vi "DisplayJson.vi"(11 "JSON String In":string="[{\"version\":\"1.0.0\",\"header\":{\"creationDate\":\"2022-06-03T00:00:00\",\"remarks\":\"\",\"serialNumber\":\"98172\",\"productNumber\":\"123021.1804\",\"productType\":\"PAA-9L\",\"pressureType\":2,\"productSeries\":\"9L\",\"compensatedTemperatureRange\":{\"min\":-10.0,\"max\":80.0,\"unit\":4},\"compensatedPressureRange\":{\"min\":0.0,\"max\":0.35,\"unit\":3},\"electricSupply\":{\"magnitude\":1.0,\"unit\":18},\"orderNumber\":9990266,\"orderPosition\":3,\"orderTargetDispatchDate\":\"2022-06-02T00:00:00+00:00\",\"customerName\":\"DemoData Inc.\",\"customerNumber\":12345678,\"customerOrderNumber\":\"Cust-9990266-123\",\"customerReferenceNumber\":\"\",\"customerProductT...") -> ()   [LabVIEW 2017] (continued)
output\":{\"magnitude\":0.109965,\"unit\":3},\"error\":{\"magnitude\":-0.0092906517,\"unit\":7}},\"temperature\":{\"output\":{\"magnitude\":19.5444,\"unit\":4},\"error\":{\"magnitude\":-0.0064905507,\"unit\":4}}}}}},{\"reference\":\"F_12300_XX_0000098765\",\"environmentTarget\":{\"pressure\":{\"magnitude\":0.19,\"unit\":3},\"temperature\":{\"magnitude\":20.0,\"unit\":4}},\"environment\":{\"pressure\":{\"magnitude\":0.190006,\"unit\":3},\"temperature\":{\"magnitude\":19.5509,\"unit\":4},\"supply\":{\"magnitude\":1.0,\"unit\":18}},\"raw\":{\"signal\":{\"magnitude\":42.078711244,\"unit\":22},\"bridgeResistance\":{\"magnitude\":3496.1789897,\"unit\":28}},\"compensated\":{\"mathematicalModels\":{\"MM0123\":{\"pressure\":{\"output\":{\"magnitude\":0.190012,\"unit\":3},\"error\":{\"magnitude\":0.0015735789,\"unit\":7}},\"temperature\":{\"output\":{\"magnitude\":19.544,\"unit\":4},\"error\":{\"magnitude\":-0.0068909382,\"unit\":4}}}}}},{\"reference\":\"F_12300_XX_0000098765\",\"environmentTarget\":{\"pressure\":{\"magnitude\":0.27,\"unit\":3},\"temperature\":{\"magnitude\":20.0,\"unit\":4}},\"environment\":{\"pressure\":{\"magnitude\":0.269992,\"unit\":3},\"temperature\":{\"magnitude\":19.5509,\"unit\":4},\"supply\":{\"magnitude\":1.0,\"unit\":18}},\"raw\":{\"signal\":{\"magnitude\":54.069872892,\"unit\":22},\"bridgeResistance\":{\"magnitude\":3491.6914255,\"unit\":28}},\"compensated\":{\"mathematicalModels\":{\"MM0123\":{\"pressure\":{\"output\":{\"magnitude\":0.27003,\"unit\":3},\"error\":{\"magnitude\":0.010759802,\"unit\":7}},\"temperature\":{\"output\":{\"magnitude\":19.5372,\"unit\":4},\"error\":{\"magnitude\":-0.013679718,\"unit\":4}}}}}},{\"reference\":\"F_12300_XX_0000098765\",\"environmentTarget\":{\"pressure\":{\"magnitude\":0.35,\"unit\":3},\"temperature\":{\"magnitude\":20.0,\"unit\":4}},\"environment\":{\"pressure\":{\"magnitude\":0.350007,\"unit\":3},\"temperature\":{\"magnitude\":19.5509,\"unit\":4},\"supply\":{\"magnitude\":1.0,\"unit\":18}},\"raw\":{\"signal\":{\"magnitude\":66.008929835,\"unit\":22},\"bridgeResistance\":{\"magnitude\":3487.3457136,\"unit\":28}},\"compensated\":{\"mathematicalModels\":{\"MM0123\":{\"pressure\":{\"output\":{\"magnitude\":0.350006,\"unit\":3},\"error\":{\"magnitude\":-0.00038101157,\"unit\":7}},\"temperature\":{\"output\":{\"magnitude\":19.5357,\"unit\":4},\"error\":{\"magnitude\":-0.015189517,\"unit\":4}}}}}},{\"reference\":\"F_12300_XX_0000098765\",\"environmentTarget\":{\"pressure\":{\"magnitude\":0.03,\"unit\":3},\"temperature\":{\"magnitude\":40.0,\"unit\":4}},\"environment\":{\"pressure\":{\"magnitude\":0.0299915,\"unit\":3},\"temperature\":{\"magnitude\":39.7284,\"unit\":4},\"supply\":{\"magnitude\":1.0,\"unit\":18}},\"raw\":{\"signal\":{\"magnitude\":19.022094163,\"unit\":22},\"bridgeResistance\":{\"magnitude\":3681.6183819,\"unit\":28}},\"compensated\":{\"mathematicalModels\":{\"MM0123\":{\"pressure\":{\"output\":{\"magnitude\":0.0300123,\"unit\":3},\"error\":{\"magnitude\":0.0059539043,\"unit\":7}},\"temperature\":{\"output\":{\"magnitude\":39.719,\"unit\":4},\"error\":{\"magnitude\":-0.0093796899,\"unit\":4}}}}}},{\"reference\":\"F_12300_XX_0000098765\",\"environmentTarget\":{\"pressure\":{\"magnitude\":0.11,\"unit\":3},\"temperature\":{\"magnitude\":40.0,\"unit\":4}},\"environment\":{\"pressure\":{\"magnitude\":0.110003,\"unit\":3},\"temperature\":{\"magnitude\":39.7284,\"unit\":4},\"supply\":{\"magnitude\":1.0,\"unit\":18}},\"raw\":{\"signal\":{\"magnitude\":31.15514702,\"unit\":22},\"bridgeResistance\":{\"magnitude\":3676.9975385,\"unit\":28}},\"compensated\":{\"mathematicalModels\":{\"MM0123\":{\"pressure\":{\"output\":{\"magnitude\":0.109971,\"unit\":3},\"error\":{\"magnitude\":-0.0090594959,\"unit\":7}},\"temperature\":{\"output\":{\"magnitude\":39.7198,\"unit\":4},\"error\":{\"magnitude\":-0.0086481985,\"unit\":4}}}}}},{\"reference\":\"F_12300_XX_0000098765\",\"environmentTarget\":{\"pressure\":{\"magnitude\":0.19,\"unit\":3},\"temperature\":{\"magnitude\":40.0,\"unit\":4}},\"environment\":{\"pressure\":{\"magnitude\":0.190008,\"unit\":3},\"temperature\":{\"magnitude\":39.7284,\"unit\":4},\"supply\":{\"magnitude\":1.0,\"unit\":18}},\"raw\":{\"signal\":{\"magnitude\":43.258033725,\"unit\":22},\"bridgeResistance\":{\"magnitude\":3672.3845946,\"unit\":28}},\"compensated\":{\"mathematicalModels\":{\"MM0123\":{\"pressure\":{\"output\":{\"magnitude\":0.190008,\"unit\":3},\"error\":{\"magnitude\":1.3837864E-05,\"unit\":7}},\"temperature\":{\"output\":{\"magnitude\":39.7143,\"unit\":4},\"error\":{\"magnitude\":-0.014086538,\"unit\":4}}}}}},{\"reference\":\"F_12300_XX_0000098765\",\"environmentTarget\":{\"pressure\":{\"magnitude\":0.27,\"unit\":3},\"temperature\":{\"magnitude\":40.0,\"unit\":4}},\"environment\":{\"pressure\":{\"magnitude\":0.269997,\"unit\":3},\"temperature\":{\"magnitude\":39.7284,\"unit\":4},\"supply\":{\"magnitude\":1.0,\"unit\":18}},\"raw\":{\"signal\":{\"magnitude\":55.315656363,\"unit\":22},\"bridgeResistance\":{\"magnitude\":3667.8577878,\"unit\":28}},\"compensated\":{\"mathematicalModels\":{\"MM0123\":{\"pressure\":{\"output\":{\"magnitude\":0.27002,\"unit\":3},\"error\":{\"magnitude\":0.006463758,\"unit\":7}},\"temperature\":{\"output\":{\"magnitude\":39.7105,\"unit\":4},\"error\":{\"magnitude\":-0.01792275,\"unit\":4}}}}}},{\"reference\":\"F_12300_XX_0000098765\",\"environmentTarget\":{\"pressure\":{\"magnitude\":0.35,\"unit\":3},\"temperature\":{\"magnitude\":40.0,\"unit\":4}},\"environment\":{\"pressure\":{\"magnitude\":0.349999,\"unit\":3},\"temperature\":{\"magnitude\":39.7284,\"unit\":4},\"supply\":{\"magnitude\":1.0,\"unit\":18}},\"raw\":{\"signal\":{\"magnitude\":67.323949938,\"unit\":22},\"bridgeResistance\":{\"magnitude\":3663.4696819,\"unit\":28}},\"compensated\":{\"mathematicalModels\":{\"MM0123\":{\"pressure\":{\"output\":{\"magnitude\":0.349975,\"unit\":3},\"error\":{\"magnitude\":-0.0067658595,\"unit\":7}},\"temperature\":{\"output\":{\"magnitude\":39.7137,\"unit\":4},\"error\":{\"magnitude\":-0.014709374,\"unit\":4}}}}}},{\"reference\":\"F_12300_XX_0000098765\",\"environmentTarget\":{\"pressure\":{\"magnitude\":0.03,\"unit\":3},\"temperature\":{\"magnitude\":60.0,\"unit\":4}},\"environment\":{\"pressure\":{\"magnitude\":0.030001,\"unit\":3},\"temperature\":{\"magnitude\":59.8651,\"unit\":4},\"supply\":{\"magnitude\":1.0,\"unit\":18}},\"raw\":{\"signal\":{\"magnitude\":20.199212253,\"unit\":22},\"bridgeResistance\":{\"magnitude\":3874.0547528,\"unit\":28}},\"compensated\":{\"mathematicalModels\":{\"MM0123\":{\"pressure\":{\"output\":{\"magnitude\":0.030016,\"unit\":3},\"error\":{\"magnitude\":0.0042926398,\"unit\":7}},\"temperature\":{\"output\":{\"magnitude\":59.9326,\"unit\":4},\"error\":{\"magnitude\":0.067505354,\"unit\":4}}}}}},{\"reference\":\"F_12300_XX_0000098765\",\"environmentTarget\":{\"pressure\":{\"magnitude\":0.11,\"unit\":3},\"temperature\":{\"magnitude\":60.0,\"unit\":4}},\"environment\":{\"pressure\":{\"magnitude\":0.110002,\"unit\":3},\"temperature\":{\"magnitude\":59.8651,\"unit\":4},\"supply\":{\"magnitude\":1.0,\"unit\":18}},\"raw\":{\"signal\":{\"magnitude\":32.429468946,\"unit\":22},\"bridgeResistance\":{\"magnitude\":3869.345801,\"unit\":28}},\"compensated\":{\"mathematicalModels\":{\"MM0123\":{\"pressure\":{\"output\":{\"magnitude\":0.109968,\"unit\":3},\"error\":{\"magnitude\":-0.0097852459,\"unit\":7}},\"temperature\":{\"output\":{\"magnitude\":59.9341,\"unit\":4},\"error\":{\"magnitude\":0.068990286,\"unit\":4}}}}}},{\"reference\":\"F_12300_XX_0000098765\",\"environmentTarget\":{\"pressure\":{\"magnitude\":0.19,\"unit\":3},\"temperature\":{\"magnitude\":60.0,\"unit\":4}},\"environment\":{\"pressure\":{\"magnitude\":0.189998,\"unit\":3},\"temperature\":{\"magnitude\":59.8651,\"unit\":4},\"supply\":{\"magnitude\":1.0,\"unit\":18}},\"raw\":{\"signal\":{\"magnitude\":44.635667683,\"unit\":22},\"bridgeResistance\":{\"magnitude\":3864.7229343,\"unit\":28}},\"compensated\":{\"mathematicalModels\":{\"MM0123\":{\"pressure\":{\"output\":{\"magnitude\":0.190005,\"unit\":3},\"error\":{\"magnitude\":0.0019461489,\"unit\":7}},\"temperature\":{\"output\":{\"magnitude\":59.9385,\"unit\":4},\"error\":{\"magnitude\":0.073372389,\"unit\":4}}}}}},{\"reference\":\"F_12300_XX_0000098765\",\"environmentTarget\":{\"pressure\":{\"magnitude\":0.27,\"unit\":3},\"temperature\":{\"magnitude\":60.0,\"unit\":4}},\"environment\":{\"pressure\":{\"magnitude\":0.270006,\"unit\":3},\"temperature\":{\"magnitude\":59.8651,\"unit\":4},\"supply\":{\"magnitude\":1.0,\"unit\":18}},\"raw\":{\"signal\":{\"magnitude\":56.803223239,\"unit\":22},\"bridgeResistance\":{\"magnitude\":3860.1295265,\"unit\":28}},\"compensated\":{\"mathematicalModels\":{\"MM0123\":{\"pressure\":{\"output\":{\"magnitude\":0.270035,\"unit\":3},\"error\":{\"magnitude\":0.0082031389,\"unit\":7}},\"temperature\":{\"output\":{\"magnitude\":59.9395,\"unit\":4},\"error\":{\"magnitude\":0.074382902,\"unit\":4}}}}}},{\"reference\":\"F_12300_XX_0000098765\",\"environmentTarget\":{\"pressure\":{\"magnitude\":0.35,\"unit\":3},\"temperature\":{\"magnitude\":60.0,\"unit\":4}},\"environment\":{\"pressure\":{\"magnitude\":0.349993,\"unit\":3},\"temperature\":{\"magnitude\":59.8651,\"unit\":4},\"supply\":{\"magnitude\":1.0,\"unit\":18}},\"raw\":{\"signal\":{\"magnitude\":68.921120737,\"unit\":22},\"bridgeResistance\":{\"magnitude\":3855.6216292,\"unit\":28}},\"compensated\":{\"mathematicalModels\":{\"MM0123\":{\"pressure\":{\"output\":{\"magnitude\":0.349982,\"unit\":3},\"error\":{\"magnitude\":-0.0031971685,\"unit\":7}},\"temperature\":{\"output\":{\"magnitude\":59.9424,\"unit\":4},\"error\":{\"magnitude\":0.077300939,\"unit\":4}}}}}},{\"reference\":\"F_12300_XX_0000098765\",\"environmentTarget\":{\"pressure\":{\"magnitude\":0.03,\"unit\":3},\"temperature\":{\"magnitude\":80.0,\"unit\":4}},\"environment\":{\"pressure\":{\"magnitude\":0.0299933,\"unit\":3},\"temperature\":{\"magnitude\":79.9513,\"unit\":4},\"supply\":{\"magnitude\":1.0,\"unit\":18}},\"raw\":{\"signal\":{\"magnitude\":21.547294663,\"unit\":22},\"bridgeResistance\":{\"magnitude\":4081.6700258,\"unit\":28}},\"compensated\":{\"mathematicalModels\":{\"MM0123\":{\"pressure\":{\"output\":{\"magnitude\":0.0300125,\"unit\":3},\"error\":{\"magnitude\":0.005483509,\"unit\":7}},\"temperature\":{\"output\":{\"magnitude\":80.0524,\"unit\":4},\"error\":{\"magnitude\":0.10106475,\"unit\":4}}}}}},{\"reference\":\"F_12300_XX_0000098765\",\"environmentTarget\":{\"pressure\":{\"magnitude\":0.11,\"unit\":3},\"temperature\":{\"magnitude\":80.0,\"unit\":4}},\"environment\":{\"pressure\":{\"magnitude\":0.109998,\"unit\":3},\"temperature\":{\"magnitude\":79.9513,\"unit\":4},\"supply\":{\"magnitude\":1.0,\"unit\":18}},\"raw\":{\"signal\":{\"magnitude\":33.903469141,\"unit\":22},\"bridgeResistance\":{\"magnitude\":4076.9028242,\"unit\":28}},\"compensated\":{\"mathematicalModels\":{\"MM0123\":{\"pressure\":{\"output\":{\"magnitude\":0.109951,\"unit\":3},\"error\":{\"magnitude\":-0.013484717,\"unit\":7}},\"temperature\":{\"output\":{\"magnitude\":80.056,\"unit\":4},\"error\":{\"magnitude\":0.10464558,\"unit\":4}}}}}},{\"reference\":\"F_12300_XX_0000098765\",\"environmentTarget\":{\"pressure\":{\"magnitude\":0.19,\"unit\":3},\"temperature\":{\"magnitude\":80.0,\"unit\":4}},\"environment\":{\"pressure\":{\"magnitude\":0.189989,\"unit\":3},\"temperature\":{\"magnitude\":79.9513,\"unit\":4},\"supply\":{\"magnitude\":1.0,\"unit\":18}},\"raw\":{\"signal\":{\"magnitude\":46.244267152,\"unit\":22},\"bridgeResistance\":{\"magnitude\":4072.2270604,\"unit\":28}},\"compensated\":{\"mathematicalModels\":{\"MM0123\":{\"pressure\":{\"output\":{\"magnitude\":0.189994,\"unit\":3},\"error\":{\"magnitude\":0.0017968044,\"unit\":7}},\"temperature\":{\"output\":{\"magnitude\":80.065,\"unit\":4},\"error\":{\"magnitude\":0.11364392,\"unit\":4}}}}}},{\"reference\":\"F_12300_XX_0000098765\",\"environmentTarget\":{\"pressure\":{\"magnitude\":0.27,\"unit\":3},\"temperature\":{\"magnitude\":80.0,\"unit\":4}},\"environment\":{\"pressure\":{\"magnitude\":0.270002,\"unit\":3},\"temperature\":{\"magnitude\":79.9513,\"unit\":4},\"supply\":{\"magnitude\":1.0,\"unit\":18}},\"raw\":{\"signal\":{\"magnitude\":58.552894427,\"unit\":22},\"bridgeResistance\":{\"magnitude\":4067.5748697,\"unit\":28}},\"compensated\":{\"mathematicalModels\":{\"MM0123\":{\"pressure\":{\"output\":{\"magnitude\":0.27004,\"unit\":3},\"error\":{\"magnitude\":0.010741529,\"unit\":7}},\"temperature\":{\"output\":{\"magnitude\":80.0722,\"unit\":4},\"error\":{\"magnitude\":0.12089275,\"unit\":4}}}}}},{\"reference\":\"F_12300_XX_0000098765\",\"environmentTarget\":{\"pressure\":{\"magnitude\":0.35,\"unit\":3},\"temperature\":{\"magnitude\":80.0,\"unit\":4}},\"environment\":{\"pressure\":{\"magnitude\":0.349999,\"unit\":3},\"temperature\":{\"magnitude\":79.9513,\"unit\":4},\"supply\":{\"magnitude\":1.0,\"unit\":18}},\"raw\":{\"signal\":{\"magnitude\":70.812866631,\"unit\":22},\"bridgeResistance\":{\"magnitude\":4062.9569348,\"unit\":28}},\"compensated\":{\"mathematicalModels\":{\"MM0123\":{\"pressure\":{\"output\":{\"magnitude\":0.349981,\"unit\":3},\"error\":{\"magnitude\":-0.0052645095,\"unit\":7}},\"temperature\":{\"output\":{\"magnitude\":80.0778,\"unit\":4},\"error\":{\"magnitude\":0.1264479,\"unit\":4}}}}}}]},{\"version\":\"1.0.0\",\"header\":{\"creationDate\":\"2022-06-03T00:00:00\",\"remarks\":\"\",\"serialNumber\":\"98029\",\"productNumber\":\"123021.1804\",\"productType\":\"PAA-9L\",\"pressureType\":2,\"productSeries\":\"9L\",\"compensatedTemperatureRange\":{\"min\":-10.0,\"max\":80.0,\"unit\":4},\"compensatedPressureRange\":{\"min\":0.0,\"max\":0.35,\"unit\":3},\"electricSupply\":{\"magnitude\":1.0,\"unit\":18},\"orderNumber\":9990266,\"orderPosition\":3,\"orderTargetDispatchDate\":\"2022-06-02T00:00:00+00:00\",\"customerName\":\"DemoData Inc.\",\"customerNumber\":12345678,\"customerOrderNumber\":\"Cust-9990266-123\",\"customerReferenceNumber\":\"\",\"customerProductType\":\"123021-1804 Rev.AA\"},\"compensationMethods\":{\"mathematicalModels\":{\"MM0123\":{\"modelType\":\"MM0123\",\"productNumber\":\"000000.0000\",\"compensatedTemperatureRange\":{\"min\":-10.0,\"max\":80.0,\"unit\":4},\"compensatedPressureRange\":{\"min\":0.0,\"max\":0.35,\"unit\":3},\"electricSupply\":{\"magnitude\":1.0,\"unit\":18},\"parts\":{\"pressure\":{\"inputs\":[\"Sig\",\"R\"],\"output\":\"P\",\"description\":\"P = f(Sig,R)\",\"coefficients\":[[4.30391435527,-0.00440031399638,1.66896365315E-06,-2.83689839391E-10,1.80615051776E-14],[-0.136055382221,0.000146391467727,-5.60384193112E-08,9.52947074311E-12,-6.08611040973E-16],[-1.83476265264E-05,4.3796100354E-08,-2.5893067192E-11,5.98006024893E-15,-4.87217331335E-19]]},\"temperature\":{\"inputs\":[\"R\",\"Sig\"],\"output\":\"T\",\"description\":\"T = f(R,Sig)\",\"coefficients\":[[-8006.755678,-0.570294000324,-0.000242469453936],[7.89400091202,0.00176352380362,-1.43437861226E-06],[-0.00297749792856,-1.11383048589E-06,1.14192158359E-09],[5.09419214995E-07,2.6532230646E-10,-2.89169963475E-13],[-3.28903297375E-11,-2.18975763354E-14,2.42257698027E-17]]}}}}},\"measurements\":[{\"reference\":\"F_12300_XX_0000098765\",\"environmentTarget\":{\"pressure\":{\"magnitude\":0.03,\"unit\":3},\"temperature\":{\"magnitude\":-10.0,\"unit\":4}},\"environment\":{\"pressure\":{\"magnitude\":0.0300012,\"unit\":3},\"temperature\":{\"magnitude\":-10.7286,\"unit\":4},\"supply\":{\"magnitude\":1.0,\"unit\":18}},\"raw\":{\"signal\":{\"magnitude\":17.469805464,\"unit\":22},\"bridgeResistance\":{\"magnitude\":3274.3908735,\"unit\":28}},\"compensated\":{\"mathematicalModels\":{\"MM0123\":{\"pressure\":{\"output\":{\"magnitude\":0.0300128,\"unit\":3},\"error\":{\"magnitude\":0.0033214421,\"unit\":7}},\"temperature\":{\"output\":{\"magnitude\":-10.8483,\"unit\":4},\"error\":{\"magnitude\":-0.11968524,\"unit\":4}}}}}},{\"reference\":\"F_12300_XX_0000098765\",\"environmentTarget\":{\"pressure\":{\"magnitude\":0.11,\"unit\":3},\"temperature\":{\"magnitude\":-10.0,\"unit\":4}},\"environment\":{\"pressure\":{\"magnitude\":0.109989,\"unit\":3},\"temperature\":{\"magnitude\":-10.7286,\"unit\":4},\"supply\":{\"magnitude\":1.0,\"unit\":18}},\"raw\":{\"signal\":{\"magnitude\":28.6771414,\"unit\":22},\"bridgeResistance\":{\"magnitude\":3270.1197043,\"unit\":28}},\"compensated\":{\"mathematicalModels\":{\"MM0123\":{\"pressure\":{\"output\":{\"magnitude\":0.109956,\"unit\":3},\"error\":{\"magnitude\":-0.0091664382,\"unit\":7}},\"temperature\":{\"output\":{\"magnitude\":-10.8553,\"unit\":4},\"error\":{\"magnitude\":-0.12670895,\"unit\":4}}}}}},{\"reference\":\"F_12300_XX_0000098765\",\"environmentTarget\":{\"pressure\":{\"magnitude\":0.19,\"unit\":3},\"temperature\":{\"magnitude\":-10.0,\"unit\":4}},\"environment\":{\"pressure\":{\"magnitude\":0.190006,\"unit\":3},\"temperature\":{\"magnitude\":-10.7286,\"unit\":4},\"supply\":{\"magnitude\":1.0,\"unit\":18}},\"raw\":{\"signal\":{\"magnitude\":39.857823302,\"unit\":22},\"bridgeResistance\":{\"magnitude\":3266.0381919,\"unit\":28}},\"compensated\":{\"mathematicalModels\":{\"MM0123\":{\"pressure\":{\"output\":{\"magnitude\":0.190013,\"unit\":3},\"error\":{\"magnitude\":0.0018984603,\"unit\":7}},\"temperature\":{\"output\":{\"magnitude\":-10.8483,\"unit\":4},\"error\":{\"magnitude\":-0.11968275,\"unit\":4}}}}}},{\"reference\":\"F_12300_XX_0000098765\",\"environmentTarget\":{\"pressure\":{\"magnitude\":0.27,\"unit\":3},\"temperature\":{\"magnitude\":-10.0,\"unit\":4}},\"environment\":{\"pressure\":{\"magnitude\":0.27001,\"unit\":3},\"temperature\":{\"magnitude\":-10.7286,\"unit\":4},\"supply\":{\"magnitude\":1.0,\"unit\":18}},\"raw\":{\"signal\":{\"magnitude\":50.990712739,\"unit\":22},\"bridgeResistance\":{\"magnitude\":3262.0123793,\"unit\":28}},\"compensated\":{\"mathematicalModels\":{\"MM0123\":{\"pressure\":{\"output\":{\"magnitude\":0.27004,\"unit\":3},\"error\":{\"magnitude\":0.0086259919,\"unit\":7}},\"temperature\":{\"output\":{\"magnitude\":-10.8489,\"unit\":4},\"error\":{\"magnitude\":-0.12021058,\"unit\":4}}}}}},{\"reference\":\"F_12300_XX_0000098765\",\"environmentTarget\":{\"pressure\":{\"magnitude\":0.35,\"unit\":3},\"temperature\":{\"magnitude\":-10.0,\"unit\":4}},\"environment\":{\"pressure\":{\"magnitude\":0.35,\"unit\":3},\"temperature\":{\"magnitude\":-10.7286,\"unit\":4},\"supply\":{\"magnitude\":1.0,\"unit\":18}},\"raw\":{\"signal\":{\"magnitude\":62.069916782,\"unit\":22},\"bridgeResistance\":{\"magnitude\":3258.0782366,\"unit\":28}},\"compensated\":{\"mathematicalModels\":{\"MM0123\":{\"pressure\":{\"output\":{\"magnitude\":0.349995,\"unit\":3},\"error\":{\"magnitude\":-0.0013803018,\"unit\":7}},\"temperature\":{\"output\":{\"magnitude\":-10.852,\"unit\":4},\"error\":{\"magnitude\":-0.12339987,\"unit\":4}}}}}},{\"reference\":\"F_12300_XX_0000098765\",\"environmentTarget\":{\"pressure\":{\"magnitude\":0.03,\"unit\":3},\"temperature\":{\"magnitude\":0.0,\"unit\":4}},\"environment\":{\"pressure\":{\"magnitude\":0.0299969,\"unit\":3},\"temperature\":{\"magnitude\":-0.629962,\"unit\":4},\"supply\":{\"magnitude\":1.0,\"unit\":18}},\"raw\":{\"signal\":{\"magnitude\":17.964408663,\"unit\":22},\"bridgeResistance\":{\"magnitude\":3343.9011381,\"unit\":28}},\"compensated\":{\"mathematicalModels\":{\"MM0123\":{\"pressure\":{\"output\":{\"magnitude\":0.0300158,\"unit\":3},\"error\":{\"magnitude\":0.0053987776,\"unit\":7}},\"temperature\":{\"output\":{\"magnitude\":-0.757361,\"unit\":4},\"error\":{\"magnitude\":-0.12739951,\"unit\":4}}}}}},{\"reference\":\"F_12300_XX_0000098765\",\"environmentTarget\":{\"pressure\":{\"magnitude\":0.11,\"unit\":3},\"temperature\":{\"magnitude\":0.0,\"unit\":4}},\"environment\":{\"pressure\":{\"magnitude\":0.110008,\"unit\":3},\"temperature\":{\"magnitude\":-0.629962,\"unit\":4},\"supply\":{\"magnitude\":1.0,\"unit\":18}},\"raw\":{\"signal\":{\"magnitude\":29.143582019,\"unit\":22},\"bridgeResistance\":{\"magnitude\":3339.6961713,\"unit\":28}},\"compensated\":{\"mathematicalModels\":{\"MM0123\":{\"pressure\":{\"output\":{\"magnitude\":0.109982,\"unit\":3},\"error\":{\"magnitude\":-0.007512361,\"unit\":7}},\"temperature\":{\"output\":{\"magnitude\":-0.756366,\"unit\":4},\"error\":{\"magnitude\":-0.12640387,\"unit\":4}}}}}},{\"reference\":\"F_12300_XX_0000098765\",\"environmentTarget\":{\"pressure\":{\"magnitude\":0.19,\"unit\":3},\"temperature\":{\"magnitude\":0.0,\"unit\":4}},\"environment\":{\"pressure\":{\"magnitude\":0.190004,\"unit\":3},\"temperature\":{\"magnitude\":-0.629962,\"unit\":4},\"supply\":{\"magnitude\":1.0,\"unit\":18}},\"raw\":{\"signal\":{\"magnitude\":40.289309201,\"unit\":22},\"bridgeResistance\":{\"magnitude\":3335.5742298,\"unit\":28}},\"compensated\":{\"mathematicalModels\":{\"MM0123\":{\"pressure\":{\"output\":{\"magnitude\":0.190003,\"unit\":3},\"error\":{\"magnitude\":-0.00035215062,\"unit\":7}},\"temperature\":{\"output\":{\"magnitude\":-0.756538,\"unit\":4},\"error\":{\"magnitude\":-0.12657596,\"unit\":4}}}}}},{\"reference\":\"F_12300_XX_0000098765\",\"environmentTarget\":{\"pressure\":{\"magnitude\":0.27,\"unit\":3},\"temperature\":{\"magnitude\":0.0,\"unit\":4}},\"environment\":{\"pressure\":{\"magnitude\":0.269998,\"unit\":3},\"temperature\":{\"magnitude\":-0.629962,\"unit\":4},\"supply\":{\"magnitude\":1.0,\"unit\":18}},\"raw\":{\"signal\":{\"magnitude\":51.392438343,\"unit\":22},\"bridgeResistance\":{\"magnitude\":3331.5013616,\"unit\":28}},\"compensated\":{\"mathematicalModels\":{\"MM0123\":{\"pressure\":{\"output\":{\"magnitude\":0.270016,\"unit\":3},\"error\":{\"magnitude\":0.0051327146,\"unit\":7}},\"temperature\":{\"output\":{\"magnitude\":-0.763307,\"unit\":4},\"error\":{\"magnitude\":-0.13334529,\"unit\":4}}}}}},{\"reference\":\"F_12300_XX_0000098765\",\"environmentTarget\":{\"pressure\":{\"magnitude\":0.35,\"unit\":3},\"temperature\":{\"magnitude\":0.0,\"unit\":4}},\"environment\":{\"pressure\":{\"magnitude\":0.349998,\"unit\":3},\"temperature\":{\"magnitude\":-0.629962,\"unit\":4},\"supply\":{\"magnitude\":1.0,\"unit\":18}},\"raw\":{\"signal\":{\"magnitude\":62.446091822,\"unit\":22},\"bridgeResistance\":{\"magnitude\":3327.5713514,\"unit\":28}},\"compensated\":{\"mathematicalModels\":{\"MM0123\":{\"pressure\":{\"output\":{\"magnitude\":0.349968,\"unit\":3},\"error\":{\"magnitude\":-0.0085767997,\"unit\":7}},\"temperature\":{\"output\":{\"magnitude\":-0.764136,\"unit\":4},\"error\":{\"magnitude\":-0.13417397,\"unit\":4}}}}}},{\"reference\":\"F_12300_XX_0000098765\",\"environmentTarget\":{\"pressure\":{\"magnitude\":0.03,\"unit\":3},\"temperature\":{\"magnitude\":20.0,\"unit\":4}},\"environment\":{\"pressure\":{\"magnitude\":0.0300098,\"unit\":3},\"temperature\":{\"magnitude\":19.5509,\"unit\":4},\"supply\":{\"magnitude\":1.0,\"unit\":18}},\"raw\":{\"signal\":{\"magnitude\":19.016551758,\"unit\":22},\"bridgeResistance\":{\"magnitude\":3500.1401453,\"unit\":28}},\"compensated\":{\"mathematicalModels\":{\"MM0123\":{\"pressure\":{\"output\":{\"magnitude\":0.0300184,\"unit\":3},\"error\":{\"magnitude\":0.0024629145,\"unit\":7}},\"temperature\":{\"output\":{\"magnitude\":19.5448,\"unit\":4},\"error\":{\"magnitude\":-0.006076032,\"unit\":4}}}}}},{\"reference\":\"F_12300_XX_0000098765\",\"environmentTarget\":{\"pressure\":{\"magnitude\":0.11,\"unit\":3},\"temperature\":{\"magnitude\":20.0,\"unit\":4}},\"environment\":{\"pressure\":{\"magnitude\":0.109997,\"unit\":3},\"temperature\":{\"magnitude\":19.5509,\"unit\":4},\"supply\":{\"magnitude\":1.0,\"unit\":18}},\"raw\":{\"signal\":{\"magnitude\":30.183544009,\"unit\":22},\"bridgeResistance\":{\"magnitude\":3495.8738284,\"unit\":28}},\"compensated\":{\"mathematicalModels\":{\"MM0123\":{\"pressure\":{\"output\":{\"magnitude\":0.109969,\"unit\":3},\"error\":{\"magnitude\":-0.0079678298,\"unit\":7}},\"temperature\":{\"output\":{\"magnitude\":19.5361,\"unit\":4},\"error\":{\"magnitude\":-0.01481561,\"unit\":4}}}}}},{\"reference\":\"F_12300_XX_0000098765\",\"environmentTarget\":{\"pressure\":{\"magnitude\":0.19,\"unit\":3},\"temperature\":{\"magnitude\":20.0,\"unit\":4}},\"environment\":{\"pressure\":{\"magnitude\":0.189996,\"unit\":3},\"temperature\":{\"magnitude\":19.5509,\"unit\":4},\"supply\":{\"magnitude\":1.0,\"unit\":18}},\"raw\":{\"signal\":{\"magnitude\":41.325342753,\"unit\":22},\"bridgeResistance\":{\"magnitude\":3491.7607801,\"unit\":28}},\"compensated\":{\"mathematicalModels\":{\"MM0123\":{\"pressure\":{\"output\":{\"magnitude\":0.190001,\"unit\":3},\"error\":{\"magnitude\":0.0013477363,\"unit\":7}},\"temperature\":{\"output\":{\"magnitude\":19.537,\"unit\":4},\"error\":{\"magnitude\":-0.013869037,\"unit\":4}}}}}},{\"reference\":\"F_12300_XX_0000098765\",\"environmentTarget\":{\"pressure\":{\"magnitude\":0.27,\"unit\":3},\"temperature\":{\"magnitude\":20.0,\"unit\":4}},\"environment\":{\"pressure\":{\"magnitude\":0.269994,\"unit\":3},\"temperature\":{\"magnitude\":19.5509,\"unit\":4},\"supply\":{\"magnitude\":1.0,\"unit\":18}},\"raw\":{\"signal\":{\"magnitude\":52.428999284,\"unit\":22},\"bridgeResistance\":{\"magnitude\":3487.6722747,\"unit\":28}},\"compensated\":{\"mathematicalModels\":{\"MM0123\":{\"pressure\":{\"output\":{\"magnitude\":0.270027,\"unit\":3},\"error\":{\"magnitude\":0.0095039132,\"unit\":7}},\"temperature\":{\"output\":{\"magnitude\":19.5313,\"unit\":4},\"error\":{\"magnitude\":-0.019589565,\"unit\":4}}}}}},{\"reference\":\"F_12300_XX_0000098765\",\"environmentTarget\":{\"pressure\":{\"magnitude\":0.35,\"unit\":3},\"temperature\":{\"magnitude\":20.0,\"unit\":4}},\"environment\":{\"pressure\":{\"magnitude\":0.350008,\"unit\":3},\"temperature\":{\"magnitude\":19.5509,\"unit\":4},\"supply\":{\"magnitude\":1.0,\"unit\":18}},\"raw\":{\"signal\":{\"magnitude\":63.490060072,\"unit\":22},\"bridgeResistance\":{\"magnitude\":3483.7090981,\"unit\":28}},\"compensated\":{\"mathematicalModels\":{\"MM0123\":{\"pressure\":{\"output\":{\"magnitude\":0.350012,\"unit\":3},\"error\":{\"magnitude\":0.0010119697,\"unit\":7}},\"temperature\":{\"output\":{\"magnitude\":19.5308,\"unit\":4},\"error\":{\"magnitude\":-0.020086927,\"unit\":4}}}}}},{\"reference\":\"F_12300_XX_0000098765\",\"environmentTarget\":{\"pressure\":{\"magnitude\":0.03,\"unit\":3},\"temperature\":{\"magnitude\":40.0,\"unit\":4}},\"environment\":{\"pressure\":{\"magnitude\":0.0300015,\"unit\":3},\"temperature\":{\"magnitude\":39.7284,\"unit\":4},\"supply\":{\"magnitude\":1.0,\"unit\":18}},\"raw\":{\"signal\":{\"magnitude\":20.164178621,\"unit\":22},\"bridgeResistance\":{\"magnitude\":3675.6210097,\"unit\":28}},\"compensated\":{\"mathematicalModels\":{\"MM0123\":{\"pressure\":{\"output\":{\"magnitude\":0.0300153,\"unit\":3},\"error\":{\"magnitude\":0.0039506189,\"unit\":7}},\"temperature\":{\"output\":{\"magnitude\":39.7206,\"unit\":4},\"error\":{\"magnitude\":-0.0078551017,\"unit\":4}}}}}},{\"reference\":\"F_12300_XX_0000098765\",\"environmentTarget\":{\"pressure\":{\"magnitude\":0.11,\"unit\":3},\"temperature\":{\"magnitude\":40.0,\"unit\":4}},\"environment\":{\"pressure\":{\"magnitude\":0.110001,\"unit\":3},\"temperature\":{\"magnitude\":39.7284,\"unit\":4},\"supply\":{\"magnitude\":1.0,\"unit\":18}},\"raw\":{\"signal\":{\"magnitude\":31.383505326,\"unit\":22},\"bridgeResistance\":{\"magnitude\":3671.409173,\"unit\":28}},\"compensated\":{\"mathematicalModels\":{\"MM0123\":{\"pressure\":{\"output\":{\"magnitude\":0.109978,\"unit\":3},\"error\":{\"magnitude\":-0.0066409574,\"unit\":7}},\"temperature\":{\"output\":{\"magnitude\":39.7209,\"unit\":4},\"error\":{\"magnitude\":-0.0075016046,\"unit\":4}}}}}},{\"reference\":\"F_12300_XX_0000098765\",\"environmentTarget\":{\"pressure\":{\"magnitude\":0.19,\"unit\":3},\"temperature\":{\"magnitude\":40.0,\"unit\":4}},\"environment\":{\"pressure\":{\"magnitude\":0.190005,\"unit\":3},\"temperature\":{\"magnitude\":39.7284,\"unit\":4},\"supply\":{\"magnitude\":1.0,\"unit\":18}},\"raw\":{\"signal\":{\"magnitude\":42.578578407,\"unit\":22},\"bridgeResistance\":{\"magnitude\":3667.230996,\"unit\":28}},\"compensated\":{\"mathematicalModels\":{\"MM0123\":{\"pressure\":{\"output\":{\"magnitude\":0.190004,\"unit\":3},\"error\":{\"magnitude\":-0.00040952465,\"unit\":7}},\"temperature\":{\"output\":{\"magnitude\":39.7184,\"unit\":4},\"error\":{\"magnitude\":-0.010057667,\"unit\":4}}}}}},{\"reference\":\"F_12300_XX_0000098765\",\"environmentTarget\":{\"pressure\":{\"magnitude\":0.27,\"unit\":3},\"temperature\":{\"magnitude\":40.0,\"unit\":4}},\"environment\":{\"pressure\":{\"magnitude\":0.269995,\"unit\":3},\"temperature\":{\"magnitude\":39.7284,\"unit\":4},\"supply\":{\"magnitude\":1.0,\"unit\":18}},\"raw\":{\"signal\":{\"magnitude\":53.738474722,\"unit\":22},\"bridgeResistance\":{\"magnitude\":3663.1525678,\"unit\":28}},\"compensated\":{\"mathematicalModels\":{\"MM0123\":{\"pressure\":{\"output\":{\"magnitude\":0.270012,\"unit\":3},\"error\":{\"magnitude\":0.0047948546,\"unit\":7}},\"temperature\":{\"output\":{\"magnitude\":39.7196,\"unit\":4},\"error\":{\"magnitude\":-0.0089360217,\"unit\":4}}}}}},{\"reference\":\"F_12300_XX_0000098765\",\"environmentTarget\":{\"pressure\":{\"magnitude\":0.35,\"unit\":3},\"temperature\":{\"magnitude\":40.0,\"unit\":4}},\"environment\":{\"pressure\":{\"magnitude\":0.350004,\"unit\":3},\"temperature\":{\"magnitude\":39.7284,\"unit\":4},\"supply\":{\"magnitude\":1.0,\"unit\":18}},\"raw\":{\"signal\":{\"magnitude\":64.859667404,\"unit\":22},\"bridgeResistance\":{\"magnitude\":3659.0897136,\"unit\":28}},\"compensated\":{\"mathematicalModels\":{\"MM0123\":{\"pressure\":{\"output\":{\"magnitude\":0.349982,\"unit\":3},\"error\":{\"magnitude\":-0.0063797985,\"unit\":7}},\"temperature\":{\"output\":{\"magnitude\":39.7151,\"unit\":4},\"error\":{\"magnitude\":-0.013366266,\"unit\":4}}}}}},{\"reference\":\"F_12300_XX_0000098765\",\"environmentTarget\":{\"pressure\":{\"magnitude\":0.03,\"unit\":3},\"temperature\":{\"magnitude\":60.0,\"unit\":4}},\"environment\":{\"pressure\":{\"magnitude\":0.0299897,\"unit\":3},\"temperature\":{\"magnitude\":59.8651,\"unit\":4},\"supply\":{\"magnitude\":1.0,\"unit\":18}},\"raw\":{\"signal\":{\"magnitude\":21.442062511,\"unit\":22},\"bridgeResistance\":{\"magnitude\":3867.6959586,\"unit\":28}},\"compensated\":{\"mathematicalModels\":{\"MM0123\":{\"pressure\":{\"output\":{\"magnitude\":0.0300028,\"unit\":3},\"error\":{\"magnitude\":0.0040250847,\"unit\":7}},\"temperature\":{\"output\":{\"magnitude\":59.9361,\"unit\":4},\"error\":{\"magnitude\":0.070993359,\"unit\":4}}}}}},{\"reference\":\"F_12300_XX_0000098765\",\"environmentTarget\":{\"pressure\":{\"magnitude\":0.11,\"unit\":3},\"temperature\":{\"magnitude\":60.0,\"unit\":4}},\"environment\":{\"pressure\":{\"magnitude\":0.109994,\"unit\":3},\"temperature\":{\"magnitude\":59.8651,\"unit\":4},\"supply\":{\"magnitude\":1.0,\"unit\":18}},\"raw\":{\"signal\":{\"magnitude\":32.748502734,\"unit\":22},\"bridgeResistance\":{\"magnitude\":3863.4153202,\"unit\":28}},\"compensated\":{\"mathematicalModels\":{\"MM0123\":{\"pressure\":{\"output\":{\"magnitude\":0.109962,\"unit\":3},\"error\":{\"magnitude\":-0.009000343,\"unit\":7}},\"temperature\":{\"output\":{\"magnitude\":59.9368,\"unit\":4},\"error\":{\"magnitude\":0.071653366,\"unit\":4}}}}}},{\"reference\":\"F_12300_XX_0000098765\",\"environmentTarget\":{\"pressure\":{\"magnitude\":0.19,\"unit\":3},\"temperature\":{\"magnitude\":60.0,\"unit\":4}},\"environment\":{\"pressure\":{\"magnitude\":0.189995,\"unit\":3},\"temperature\":{\"magnitude\":59.8651,\"unit\":4},\"supply\":{\"magnitude\":1.0,\"unit\":18}},\"raw\":{\"signal\":{\"magnitude\":44.037696569,\"unit\":22},\"bridgeResistance\":{\"magnitude\":3859.2068092,\"unit\":28}},\"compensated\":{\"mathematicalModels\":{\"MM0123\":{\"pressure\":{\"output\":{\"magnitude\":0.190001,\"unit\":3},\"error\":{\"magnitude\":0.0016262193,\"unit\":7}},\"temperature\":{\"output\":{\"magnitude\":59.94,\"unit\":4},\"error\":{\"magnitude\":0.074845585,\"unit\":4}}}}}},{\"reference\":\"F_12300_XX_0000098765\",\"environmentTarget\":{\"pressure\":{\"magnitude\":0.27,\"unit\":3},\"temperature\":{\"magnitude\":60.0,\"unit\":4}},\"environment\":{\"pressure\":{\"magnitude\":0.270006,\"unit\":3},\"temperature\":{\"magnitude\":59.8651,\"unit\":4},\"supply\":{\"magnitude\":1.0,\"unit\":18}},\"raw\":{\"signal\":{\"magnitude\":55.297120957,\"unit\":22},\"bridgeResistance\":{\"magnitude\":3855.0156653,\"unit\":28}},\"compensated\":{\"mathematicalModels\":{\"MM0123\":{\"pressure\":{\"output\":{\"magnitude\":0.270033,\"unit\":3},\"error\":{\"magnitude\":0.007650526,\"unit\":7}},\"temperature\":{\"output\":{\"magnitude\":59.9396,\"unit\":4},\"error\":{\"magnitude\":0.074485733,\"unit\":4}}}}}},{\"reference\":\"F_12300_XX_0000098765\",\"environmentTarget\":{\"pressure\":{\"magnitude\":0.35,\"unit\":3},\"temperature\":{\"magnitude\":60.0,\"unit\":4}},\"environment\":{\"pressure\":{\"magnitude\":0.349993,\"unit\":3},\"temperature\":{\"magnitude\":59.8651,\"unit\":4},\"supply\":{\"magnitude\":1.0,\"unit\":18}},\"raw\":{\"signal\":{\"magnitude\":66.516869816,\"unit\":22},\"bridgeResistance\":{\"magnitude\":3850.924733,\"unit\":28}},\"compensated\":{\"mathematicalModels\":{\"MM0123\":{\"pressure\":{\"output\":{\"magnitude\":0.349984,\"unit\":3},\"error\":{\"magnitude\":-0.002578928,\"unit\":7}},\"temperature\":{\"output\":{\"magnitude\":59.9437,\"unit\":4},\"error\":{\"magnitude\":0.078539439,\"unit\":4}}}}}},{\"reference\":\"F_12300_XX_0000098765\",\"environmentTarget\":{\"pressure\":{\"magnitude\":0.03,\"unit\":3},\"temperature\":{\"magnitude\":80.0,\"unit\":4}},\"environment\":{\"pressure\":{\"magnitude\":0.029999,\"unit\":3},\"temperature\":{\"magnitude\":79.9513,\"unit\":4},\"supply\":{\"magnitude\":1.0,\"unit\":18}},\"raw\":{\"signal\":{\"magnitude\":22.890441738,\"unit\":22},\"bridgeResistance\":{\"magnitude\":4074.7179581,\"unit\":28}},\"compensated\":{\"mathematicalModels\":{\"MM0123\":{\"pressure\":{\"output\":{\"magnitude\":0.0300185,\"unit\":3},\"error\":{\"magnitude\":0.0055741983,\"unit\":7}},\"temperature\":{\"output\":{\"magnitude\":80.0589,\"unit\":4},\"error\":{\"magnitude\":0.10748419,\"unit\":4}}}}}},{\"reference\":\"F_12300_XX_0000098765\",\"environmentTarget\":{\"pressure\":{\"magnitude\":0.11,\"unit\":3},\"temperature\":{\"magnitude\":80.0,\"unit\":4}},\"environment\":{\"pressure\":{\"magnitude\":0.110003,\"unit\":3},\"temperature\":{\"magnitude\":79.9513,\"unit\":4},\"supply\":{\"magnitude\":1.0,\"unit\":18}},\"raw\":{\"signal\":{\"magnitude\":34.30912108,\"unit\":22},\"bridgeResistance\":{\"magnitude\":4070.3989201,\"unit\":28}},\"compensated\":{\"mathematicalModels\":{\"MM0123\":{\"pressure\":{\"output\":{\"magnitude\":0.10996,\"unit\":3},\"error\":{\"magnitude\":-0.012322445,\"unit\":7}},\"temperature\":{\"output\":{\"magnitude\":80.0628,\"unit\":4},\"error\":{\"magnitude\":0.11245703,\"unit\":4}}}}}},{\"reference\":\"F_12300_XX_0000098765\",\"environmentTarget\":{\"pressure\":{\"magnitude\":0.19,\"unit\":3},\"temperature\":{\"magnitude\":80.0,\"unit\":4}},\"environment\":{\"pressure\":{\"magnitude\":0.190001,\"unit\":3},\"temperature\":{\"magnitude\":79.9513,\"unit\":4},\"supply\":{\"magnitude\":1.0,\"unit\":18}},\"raw\":{\"signal\":{\"magnitude\":45.721004982,\"unit\":22},\"bridgeResistance\":{\"magnitude\":4066.1281108,\"unit\":28}},\"compensated\":{\"mathematicalModels\":{\"MM0123\":{\"pressure\":{\"output\":{\"magnitude\":0.190012,\"unit\":3},\"error\":{\"magnitude\":0.0031998964,\"unit\":7}},\"temperature\":{\"output\":{\"magnitude\":80.0687,\"unit\":4},\"error\":{\"magnitude\":0.11740094,\"unit\":4}}}}}},{\"reference\":\"F_12300_XX_0000098765\",\"environmentTarget\":{\"pressure\":{\"magnitude\":0.27,\"unit\":3},\"temperature\":{\"magnitude\":80.0,\"unit\":4}},\"environment\":{\"pressure\":{\"magnitude\":0.270007,\"unit\":3},\"temperature\":{\"magnitude\":79.9513,\"unit\":4},\"supply\":{\"magnitude\":1.0,\"unit\":18}},\"raw\":{\"signal\":{\"magnitude\":57.105743311,\"unit\":22},\"bridgeResistance\":{\"magnitude\":4061.91562,\"unit\":28}},\"compensated\":{\"mathematicalModels\":{\"MM0123\":{\"pressure\":{\"output\":{\"magnitude\":0.270035,\"unit\":3},\"error\":{\"magnitude\":0.0079469742,\"unit\":7}},\"temperature\":{\"output\":{\"magnitude\":80.0768,\"unit\":4},\"error\":{\"magnitude\":0.12541734,\"unit\":4}}}}}},{\"reference\":\"F_12300_XX_0000098765\",\"environmentTarget\":{\"pressure\":{\"magnitude\":0.35,\"unit\":3},\"temperature\":{\"magnitude\":80.0,\"unit\":4}},\"environment\":{\"pressure\":{\"magnitude\":0.349999,\"unit\":3},\"temperature\":{\"magnitude\":79.9513,\"unit\":4},\"supply\":{\"magnitude\":1.0,\"unit\":18}},\"raw\":{\"signal\":{\"magnitude\":68.456219384,\"unit\":22},\"bridgeResistance\":{\"magnitude\":4057.7040364,\"unit\":28}},\"compensated\":{\"mathematicalModels\":{\"MM0123\":{\"pressure\":{\"output\":{\"magnitude\":0.349983,\"unit\":3},\"error\":{\"magnitude\":-0.0044871338,\"unit\":7}},\"temperature\":{\"output\":{\"magnitude\":80.0812,\"unit\":4},\"error\":{\"magnitude\":0.12987143,\"unit\":4}}}}}}]},{\"version\":\"1.0.0\",\"header\":{\"creationDate\":\"2022-06-03T00:00:00\",\"remarks\":\"\",\"serialNumber\":\"98085\",\"productNumber\":\"123021.1804\",\"productType\":\"PAA-9L\",\"pressureType\":2,\"productSeries\":\"9L\",\"compensatedTemperatureRange\":{\"min\":-10.0,\"max\":80.0,\"unit\":4},\"compensatedPressureRange\":{\"min\":0.0,\"max\":0.35,\"unit\":3},\"electricSupply\":{\"magnitude\":1.0,\"unit\":18},\"orderNumber\":9990266,\"orderPosition\":3,\"orderTargetDispatchDate\":\"2022-06-02T00:00:00+00:00\",\"customerName\":\"DemoData Inc.\",\"customerNumber\":12345678,\"customerOrderNumber\":\"Cust-9990266-123\",\"customerReferenceNumber\":\"\",\"customerProductType\":\"123021-1804 Rev.AA\"},\"compensationMethods\":{\"mathematicalModels\":{\"MM0123\":{\"modelType\":\"MM0123\",\"productNumber\":\"000000.0000\",\"compensatedTemperatureRange\":{\"min\":-10.0,\"max\":80.0,\"unit\":4},\"compensatedPressureRange\":{\"min\":0.0,\"max\":0.35,\"unit\":3},\"electricSupply\":{\"magnitude\":1.0,\"unit\":18},\"parts\":{\"pressure\":{\"inputs\":[\"Sig\",\"R\"],\"output\":\"P\",\"description\":\"P = f(Sig,R)\",\"coefficients\":[[4.39727365012,-0.00452536345908,1.72608060703E-06,-2.94814392161E-10,1.89733516472E-14],[-0.158307547211,0.000171107372874,-6.60528990672E-08,1.1330129118E-11,-7.30019209305E-16],[0.00013080317193,-1.14679142265E-07,3.72619083413E-11,-5.20618605978E-15,2.55809442485E-19]]},\"temperature\":{\"inputs\":[\"R\",\"Sig\"],\"output\":\"T\",\"description\":\"T = f(R,Sig)\",\"coefficients\":[[-7640.9127246,-10.696562221,0.0923031671502],[7.56012879119,0.0129040023129,-0.000103514069177],[-0.00287232989768,-5.70849783919E-06,4.32835554503E-08],[4.94844718504E-07,1.1069759757E-09,-8.00582116284E-12],[-3.21812184385E-11,-7.96593584169E-14,5.53005287637E-16]]}}}}},\"measurements\":[{\"reference\":\"F_12300_XX_0000098765\",\"environmentTarget\":{\"pressure\":{\"magnitude\":0.03,\"unit\":3},\"temperature\":{\"magnitude\":-10.0,\"unit\":4}},\"environment\":{\"pressure\":{\"magnitude\":0.029999,\"unit\":3},\"temperature\":{\"magnitude\":-10.7286,\"unit\":4},\"supply\":{\"magnitude\":1.0,\"unit\":18}},\"raw\":{\"signal\":{\"magnitude\":16.195156393,\"unit\":22},\"bridgeResistance\":{\"magnitude\":3256.489958,\"unit\":28}},\"compensated\":{\"mathematicalModels\":{\"MM0123\":{\"pressure\":{\"output\":{\"magnitude\":0.0300074,\"unit\":3},\"error\":{\"magnitude\":0.0024124603,\"unit\":7}},\"temperature\":{\"output\":{\"magnitude\":-10.8255,\"unit\":4},\"error\":{\"magnitude\":-0.096822876,\"unit\":4}}}}}},{\"reference\":\"F_12300_XX_0000098765\",\"environmentTarget\":{\"pressure\":{\"magnitude\":0.11,\"unit\":3},\"temperature\":{\"magnitude\":-10.0,\"unit\":4}},\"environment\":{\"pressure\":{\"magnitude\":0.110001,\"unit\":3},\"temperature\":{\"magnitude\":-10.7286,\"unit\":4},\"supply\":{\"magnitude\":1.0,\"unit\":18}},\"raw\":{\"signal\":{\"magnitude\":26.598314112,\"unit\":22},\"bridgeResistance\":{\"magnitude\":3252.6109122,\"unit\":28}},\"compensated\":{\"mathematicalModels\":{\"MM0123\":{\"pressure\":{\"output\":{\"magnitude\":0.109978,\"unit\":3},\"error\":{\"
